vi "Write state.vi"(8 "error in (no error)":errorcluster, 10 "MountTrackStates":T1, 11 "MccRotTrack in":refnum<class "MccRotTrack.lvclass">) -> (0 "error out":errorcluster, 3 "MccRotTrack out":refnum<class "MccRotTrack.lvclass">)   [LabVIEW 2022 SP3, in "TCSDataDefinitions.lvlib" / "TCSMountControlCommand.lvlib" / "CommandsForRotatorAxis.lvlib" / "MccRotTrack.lvclass"]
uses:
  MccRotTrack.lvclass
  Enumerations/MountTrackStates.ctl
  MccRotTrack.lvclass/MccRotTrack.ctl
  TCSMountControlCommand.lvlib
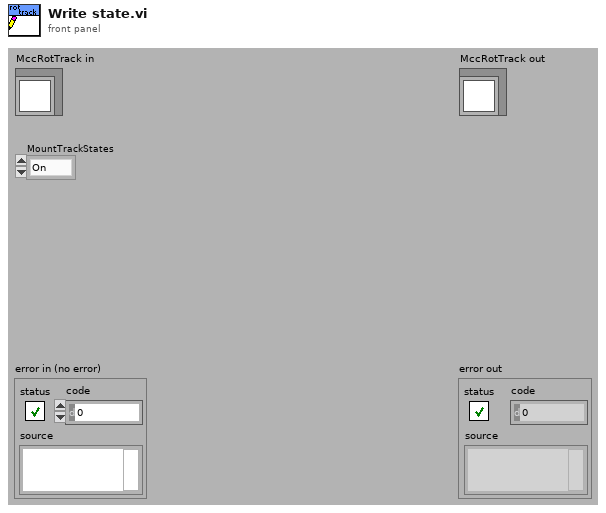
[diagram p1: front panel]
types:
  T1 = typedef "TCSDataDefinitions.lvlib/TCSMountControlCommand.lvlib/MountTrackStates.ctl" = enum16{"On", "Off"}
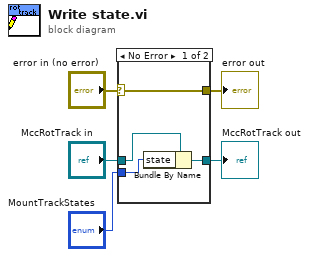
[diagram p0: block diagram]
diagram:
  n1 = case shown="No Error" "error in (no error)" {
    selector: "error in (no error)" -> [w9 w10]
    tunnel: [w9 w10] -> w4
    tunnel: [w7 w11] -> w2
    tunnel: "MccRotTrack in" -> [w8 w11]
    tunnel: "MountTrackStates" -> [w6 _]
    frame No Error {
      n2 = Bundle By Name(cluster=w8, "state"=w6) -> (w7:refnum<class "MccRotTrack.lvclass">)
    }
    frame Error {
    }
  }
  "error out" <- w4
  "MccRotTrack out" <- w2
